vi "GetData (1).vi"(11 "Tag":string="test") -> (1 "Numeric":dbl)   [LabVIEW 2018]
uses:
  subs/SLC_Types.ctl
  <vilib>/httpClient/LabVIEWHTTPClient.lvlib
panel:
  in  "stop":bool
  # "If you do not wire anything into Value In,\nLabVIEW will convert the Numeric in into a\nstring and send that."
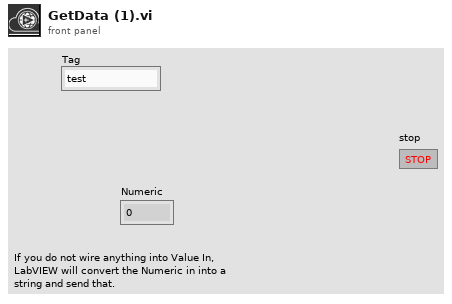
[diagram p1: front panel]
types:
  T1 = typedef "SLC_Types.ctl" = string
  T2 = typedef "LabVIEWHTTPClient.lvlib/ClientHandle.ctl" = refnum<k1>
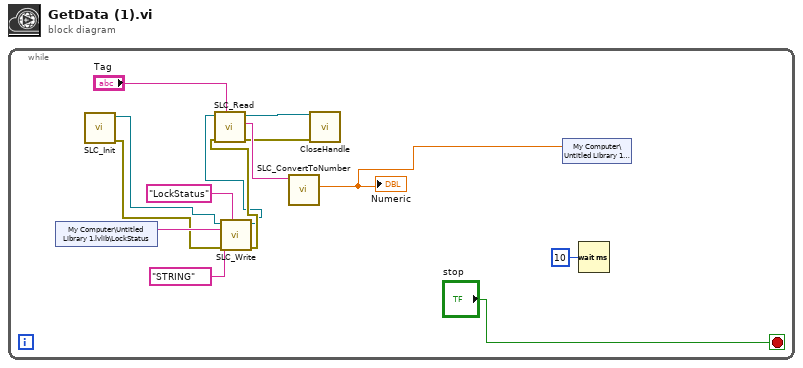
[diagram p0: block diagram]
diagram:
  n1 = while {
    stop <- "stop" stop-if-true
    n2 = shared-variable "My Computer\\Untitled Library 1.lvlib\\LockStatus"() -> (w8:string)  [unwired: 1 in, 1 out]
    n3 = call "SLC_Init.vi"() -> ("error out"=w6:errorcluster, "Refnum out"=w4:T2)  [unwired: 10 in]
    n4 = call "SLC_Write.vi"("Tag"="LockStatus", "error in"=w6, "Type"=T1 "STRING", "Write String"=w8, "Refnum in"=w4) -> ("error out"=w5:errorcluster, "Refnum out"=w3:T2)  [unwired: 3 in, 2 out]
    n5 = call "SLC_Read.vi"("Tag"="Tag", "error in"=w5, "Refnum in"=w3) -> ("error out"=w12:errorcluster, "body"=w14:string, "Refnum out"=w13:T2)  [unwired: 5 in, 1 out]
    n6 = call "SLC_ConvertToNumber.vi"("body"=w14) -> ("Numeric"=w10:dbl)  [unwired: 8 in, 2 out]
    "Numeric" <- w10
    n7 = call <vilib>:"CloseHandle.vi"("client handle"=w13, "error in (no error)"=w12) -> ()  [unwired: 13 in, 1 out]
    n8 = shared-variable "My Computer\\Untitled Library 1.lvlib\\RFID"(w10) -> ()  [unwired: 1 in, 1 out]
    n9 = Wait (ms)(milliseconds to wait=u32 10) -> ()  [unwired: 1 out]
  }
